vi "CenterBack.vi"(0 "Our Robot in":T3={"id"=0, "function"=enum."Attacker", "x"=0.0, "y"=0.0, "orientation"=0.0, "v_tangent"=0.0, "v_normal"=0.0, "v_ang"=0.0, "kick_x"=0.0, "kick_z"=0.0, "dribble"=FALSE, "Timestamp"=timestamp(0 s since 1904-01-01), "estimatives"={"est_v_tangent"=0.0, "est_v_normal"=0.0, "est_vx"=0.0, "est_vy"=0.0, "Pos Robot Est"=[]}, "dest_x_kick"=0.0, "dest_y_kick"=0.0, "Gap Coord"=[], "States"=enum."GoToTangent", "Path "=[], "Path  Smooth"=[], "Dest"=[]}, 1 "total":i32, 2 "Id duelist":u32, 3 "Stop?":bool, 4 "AI Parameters":T1={"GotoKick"={"Dist do cone a frente"=150.0, "attacker farback"=1500.0, "Perto"=300.0, "min dist to kick"=150.0, "kick eps"=0.05, "Time to transition"=0.0}, "Attacker"={"CC chute"=0.09, "CC passe"=0.045, "Kick Force"=100.0, "ball-robot Kick"=200.0, "ball-robot Pass"=0.3, "drible\nAttk"=FALSE}, "Defender"={"D max"=1700.0, "Vel p/ robô av"=1000.0, "Kick Force"=100.0, "D atk-def"=0.0, "D farback"=0.0, "drible\ndef"=FALSE, "drible\ngoalie"=FALSE}, "Timeout"={"Field/v in x"=6.0, "Dist Robots"=300, "Dist up in y"=300}, "Pose Striker"={"dist"=200.0, "Numeric"=-4.0, "dist 2"=200.0, "drible\nstriker"=FALSE}, "Dist Stop"=300.0, "D ball out"=200, "D central gap "=150.0, "T pass"=0.0, "Force ++"=0.0, "range kick"=0.0, "Chute alto"=TRUE, "Marcador novo"=TRUE, "drible"=FALSE, "D drible"=300.0} {"D drible" format="%#_13g"; "D central gap" format="%#_13g"; "Dist Stop" format="%#_13g"; "Pose Striker"."Numeric" format="%#_13g"; "Defender"."Kick Force" format="%#_13g"; "Defender"."Vel p/ robô av" format="%#_13g"; "Attacker"."ball-robot Kick" format="%#_13g"; "Attacker"."Kick Force" format="%#_13g"; "Attacker"."CC passe" format="%#_13g"; "Attacker"."CC chute" format="%#_13g"; "GotoKick"."kick eps" format="%#_13g"; "GotoKick"."min dist to kick" format="%#_13g"; "GotoKick"."Perto" format="%#_13g"; "GotoKick"."attacker farback" format="%#_13g"; "GotoKick"."Dist do cone a frente" format="%#_13g"}, 5 "balls":T8[](array[typedef]), 7 "Dribble":bool=TRUE, 9 "Field Size in":T9, 10 "Atacando contra?":bool=TRUE, 11 "Field defense":dbl[](array[numeric]), 12 "Defensores":u32[](array[numeric]), 14 "IA State Input 2":T2={"our_robots"=[], "enemy_robots"=[], "balls"=[], "geometry"={"line_width"=0, "field_length"=0, "field_width"=0, "boundary_width"=0, "referee_width"=0, "goal_width"=0, "goal_depth"=0, "goal_wall_width"=0, "center_circle_radius"=0, "defense_radius"=0, "defense_stretch"=0, "free_kick_from_defense_dist"=0, "penalty_spot_from_field_line_dist"=0, "penalty_line_from_spot_dist"=0}, "IA Judge"={"stage"="", "command"="", "our_goalie_id"=0.0, "enemy_goalie_id"=0.0, "command enum"=enum."Halt", "Time"=enum."Azul"}, "Received Timestamp"=timestamp(0 s since 1904-01-01), "Events"={"Touch"=FALSE, "Ball out"=FALSE, "id touch"=0.0, "Ball out of \nVision"=FALSE, "Ball inside \nGoalie area"=FALSE, "Robot not responding"=FALSE, "Robots responding status"=[1.0, 1.0, 1.0, 1.0, 1.0, 1.0], "Enemy Ball \nPossession"=FALSE, "Pass State"=FALSE, "id end of pass"=0.0, "Kick"=FALSE, "Id ini Possession"=0.0, "Ball Possesion"=FALSE, "Id Possesion"=0.0}}) -> (6 "Robot out":T3={"id"=0, "function"=enum."Attacker", "x"=0.0, "y"=0.0, "orientation"=0.0, "v_tangent"=0.0, "v_normal"=0.0, "v_ang"=0.0, "kick_x"=0.0, "kick_z"=0.0, "dribble"=FALSE, "Timestamp"=timestamp(0 s since 1904-01-01), "estimatives"={"est_v_tangent"=0.0, "est_v_normal"=0.0, "est_vx"=0.0, "est_vy"=0.0, "Pos Robot Est"=[]}, "dest_x_kick"=0.0, "dest_y_kick"=0.0, "Gap Coord"=[], "States"=enum."GoToTangent", "Path "=[], "Path  Smooth"=[], "Dest"=[]}, 8 "Pos Centers Back":dbl[][](array[numeric]), 13 "Zageuiro duelist?":bool=TRUE)   [LabVIEW 2017]
uses:
  Core/AI Robot.ctl
  Functions Enum.ctl
  AttackerStates.ctl
  Path Planning/RRT/PathDests.ctl
  Path Planning/RRT/PathDest.ctl
  Core/AI Ball.ctl
  Core/Field Size.ctl
  Core/AI Input.ctl
  Core/AI Judge.ctl
  Command Enum.ctl
  Util/Events/Events.ctl
  AI Parameters.ctl
  PersonalityEnum.ctl
  <vilib>/Analysis/_algsub.llb/Real Vector Norm.vi
  <vilib>/Analysis/NI_AALPro.lvlib
panel:
  in  "element":dbl=-2000.0 format="%#_13g"
  in  "dist to defender\nattacker evasion":dbl=200.0
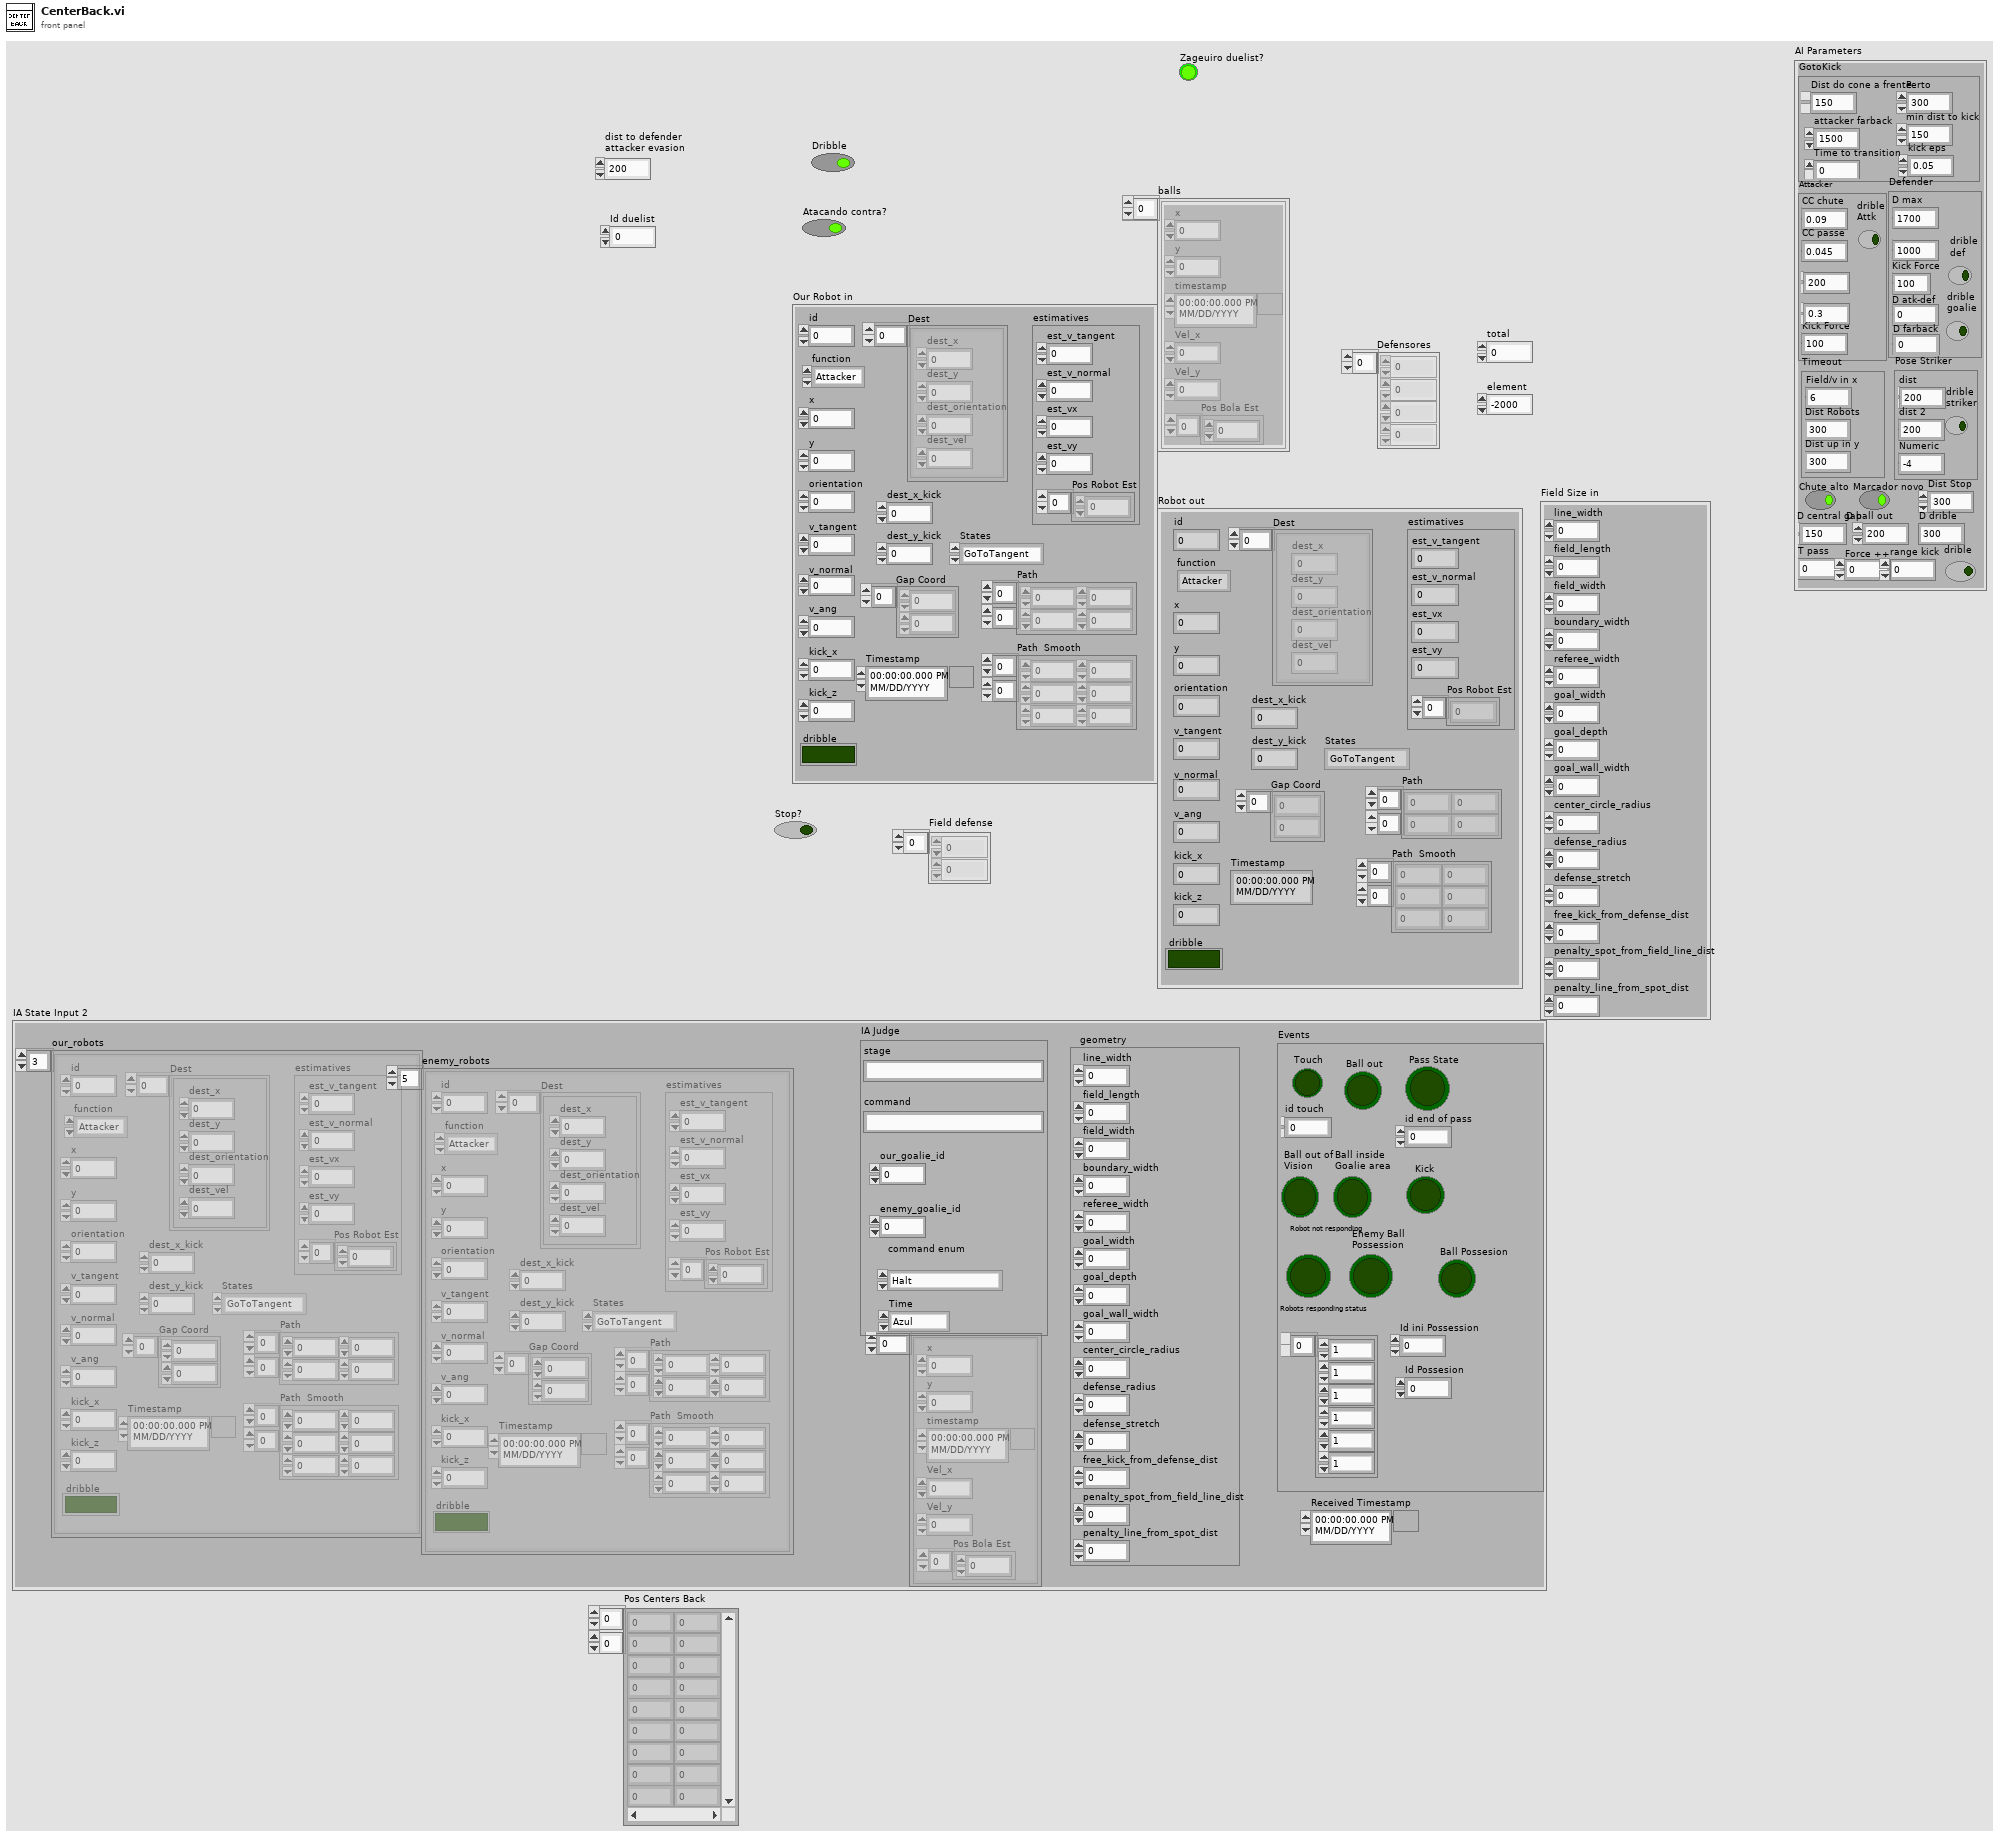
[diagram p1: front panel]
types:
  T1 = typedef "AI Parameters.ctl" = cluster{"GotoKick":cluster{"Dist do cone a frente":dbl, "attacker farback":dbl, "Perto":dbl, "min dist to kick":dbl, "kick eps":dbl, "Time to transition":dbl}, "Attacker":cluster{"CC chute":dbl, "CC passe":dbl, "Kick Force":dbl, "ball-robot Kick":dbl, "ball-robot Pass":dbl, "drible\nAttk":bool}, "Defender":cluster{"D max":dbl, "Vel p/ robô av":dbl, "Kick Force":dbl, "D atk-def":dbl, "D farback":dbl, "drible\ndef":bool, "drible\ngoalie":bool}, "Timeout":cluster{"Field/v in x":dbl, "Dist Robots":u32, "Dist up in y":u32}, "Pose Striker":cluster{"dist":dbl, "Numeric":dbl, "dist 2":dbl, "drible\nstriker":bool}, "Dist Stop":dbl, "D ball out":i32, "D central gap ":dbl, "T pass":dbl, "Force ++":dbl, "range kick":dbl, "Chute alto":bool, "Marcador novo":bool, "drible":bool, "D drible":dbl}
  T2 = typedef "AI Input.ctl" = cluster{"our_robots":T3[], "enemy_robots":T3[], "balls":T8[], "geometry":T9, "IA Judge":T10, "Received Timestamp":timestamp, "Events":T12}
  T3 = typedef "AI Robot.ctl" = cluster{"id":u32, "function":T4, "x":dbl, "y":dbl, "orientation":dbl, "v_tangent":dbl, "v_normal":dbl, "v_ang":dbl, "kick_x":dbl, "kick_z":dbl, "dribble":bool, "Timestamp":timestamp, "estimatives":cluster{"est_v_tangent":dbl, "est_v_normal":dbl, "est_vx":dbl, "est_vy":dbl, "Pos Robot Est":dbl[]}, "dest_x_kick":dbl, "dest_y_kick":dbl, "Gap Coord":dbl[], "States":T5, "Path ":dbl[][], "Path  Smooth":dbl[][], "Dest":T6}
  T4 = typedef "Functions Enum.ctl" = enum16{"Attacker", "Goalie", "Defender", "Striker", "Goto 0", "Dummy", "Kicker", "ZigZag"}
  T5 = typedef "AttackerStates.ctl" = enum16{"Pass", "GoToTangent", "BallGetting", "GoToKick", ""}
  T6 = typedef "PathDests.ctl" = T7[]
  T7 = typedef "PathDest.ctl" = cluster{"dest_x":dbl, "dest_y":dbl, "dest_orientation":dbl, "dest_vel":dbl}
  T8 = typedef "AI Ball.ctl" = cluster{"x":dbl, "y":dbl, "timestamp":timestamp, "Vel_x":dbl, "Vel_y":dbl, "Pos Bola Est":dbl[]}
  T9 = typedef "Field Size.ctl" = cluster{"line_width":u32, "field_length":u32, "field_width":u32, "boundary_width":u32, "referee_width":u32, "goal_width":u32, "goal_depth":u32, "goal_wall_width":u32, "center_circle_radius":u32, "defense_radius":u32, "defense_stretch":u32, "free_kick_from_defense_dist":u32, "penalty_spot_from_field_line_dist":u32, "penalty_line_from_spot_dist":u32}
  T10 = typedef "AI Judge.ctl" = cluster{"stage":string, "command":string, "our_goalie_id":dbl, "enemy_goalie_id":dbl, "command enum":T11, "Time":enum16{"Azul", "Amarelo"}}
  T11 = typedef "Command Enum.ctl" = enum16{"Halt", "Stop", "Force Start", "PKA Normal Start", "Prepare Kickoff Ally", "PKE Normal Start", "Prepare Kickoff Enemy", "Prepare Penalty Ally", "PPA Normal Start", "Prepare Penalty Enemy", "PPE Normal Start", "Direct Free Enemy", "Direct Free Ally", "Indirect Free Enemy", "Indirect Free Ally", "Timeout Enemy", "Timeout Ally", "Goal Enemy", "Goal Ally", "Ball Placement Enemy", "Ball Placement Ally", "Normal Half Time", "Extra Time Break", "Extra Half Time", "None", "Post Game"}
  T12 = typedef "Events.ctl" = cluster{"Touch":bool, "Ball out":bool, "id touch":dbl, "Ball out of \nVision":bool, "Ball inside \nGoalie area":bool, "Robot not responding":bool, "Robots responding status":dbl[], "Enemy Ball \nPossession":bool, "Pass State":bool, "id end of pass":dbl, "Kick":bool, "Id ini Possession":dbl, "Ball Possesion":bool, "Id Possesion":dbl}
  T13 = cluster{"D max":dbl, "Vel p/ robô av":dbl, "Kick Force":dbl, "D atk-def":dbl, "D farback":dbl, "drible\ndef":bool, "drible\ngoalie":bool}
  T14 = typedef "PersonalityEnum.ctl" = enum16{"Attacker", "Striker", "Defender", "Goalie"}
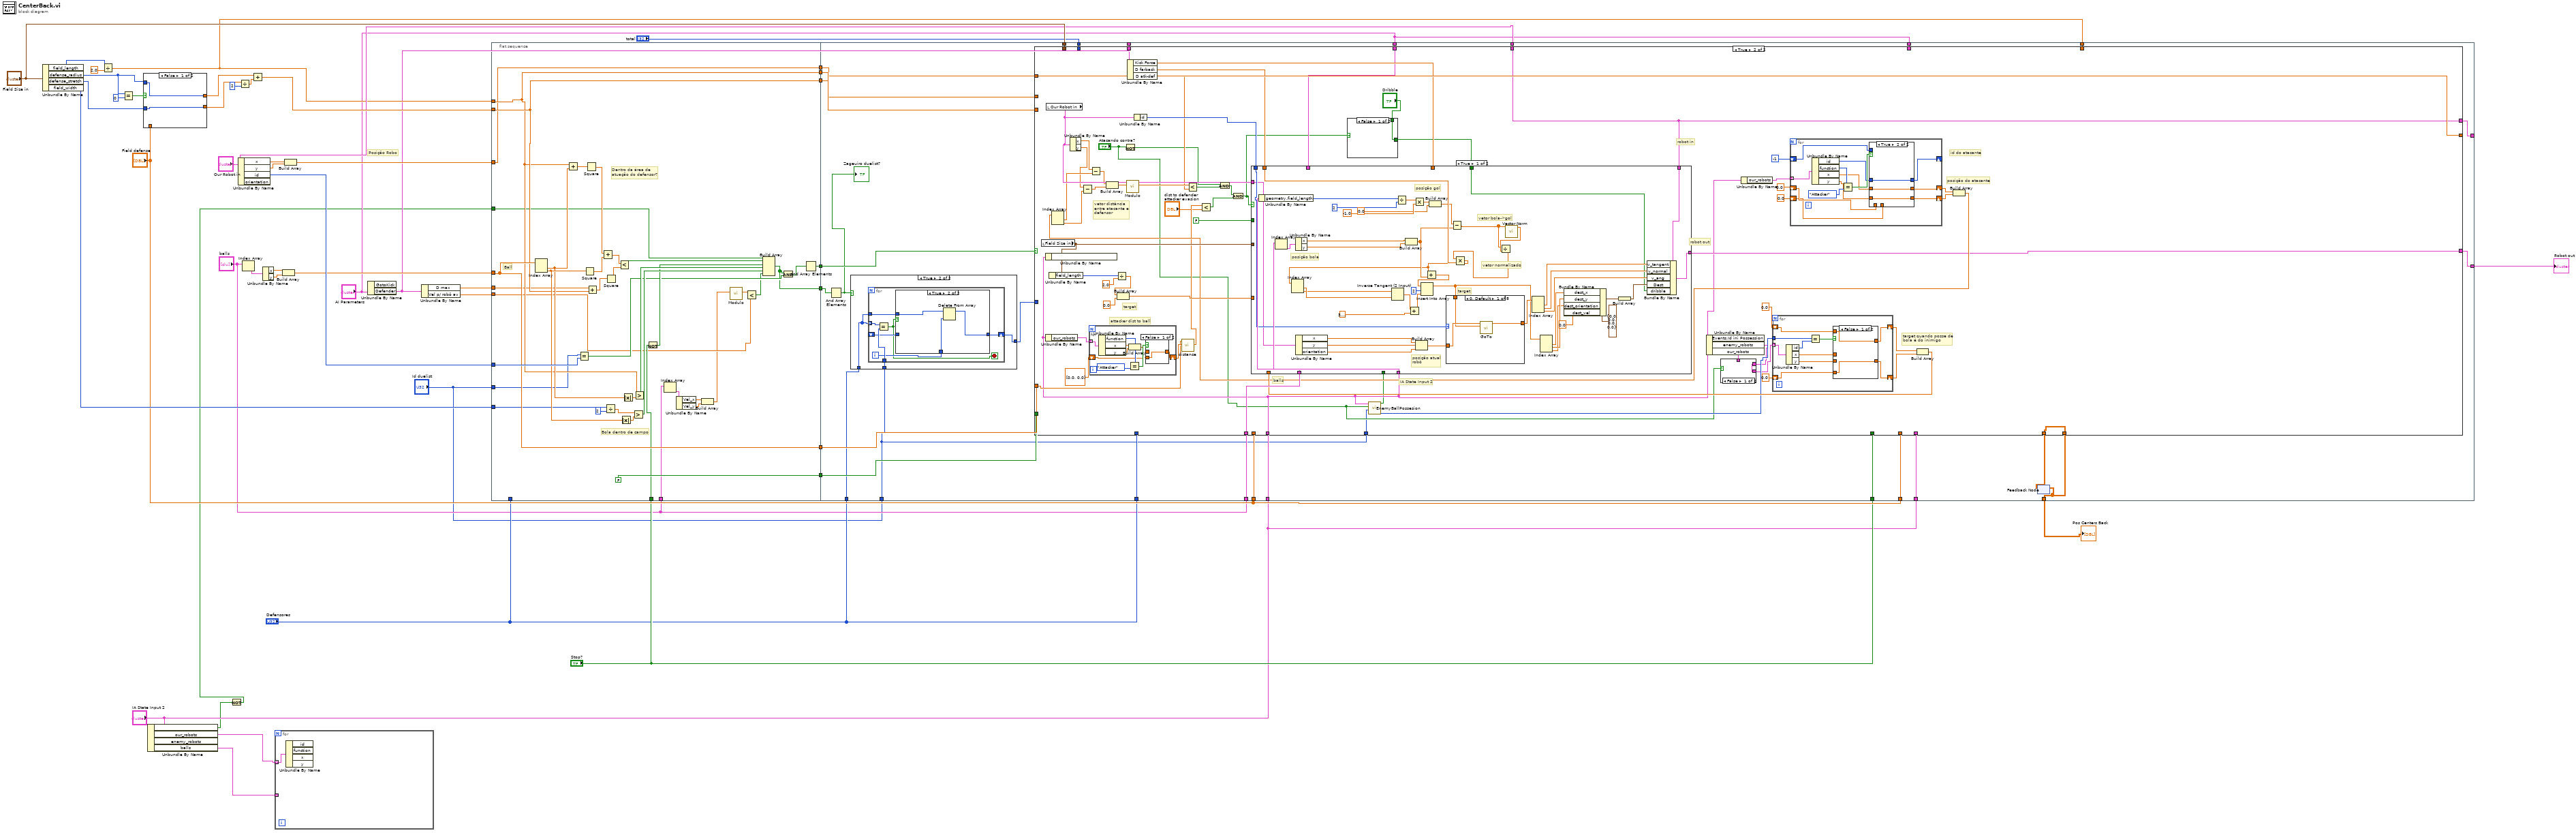
[diagram p0: block diagram]
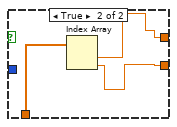
[diagram p2: hidden frame]
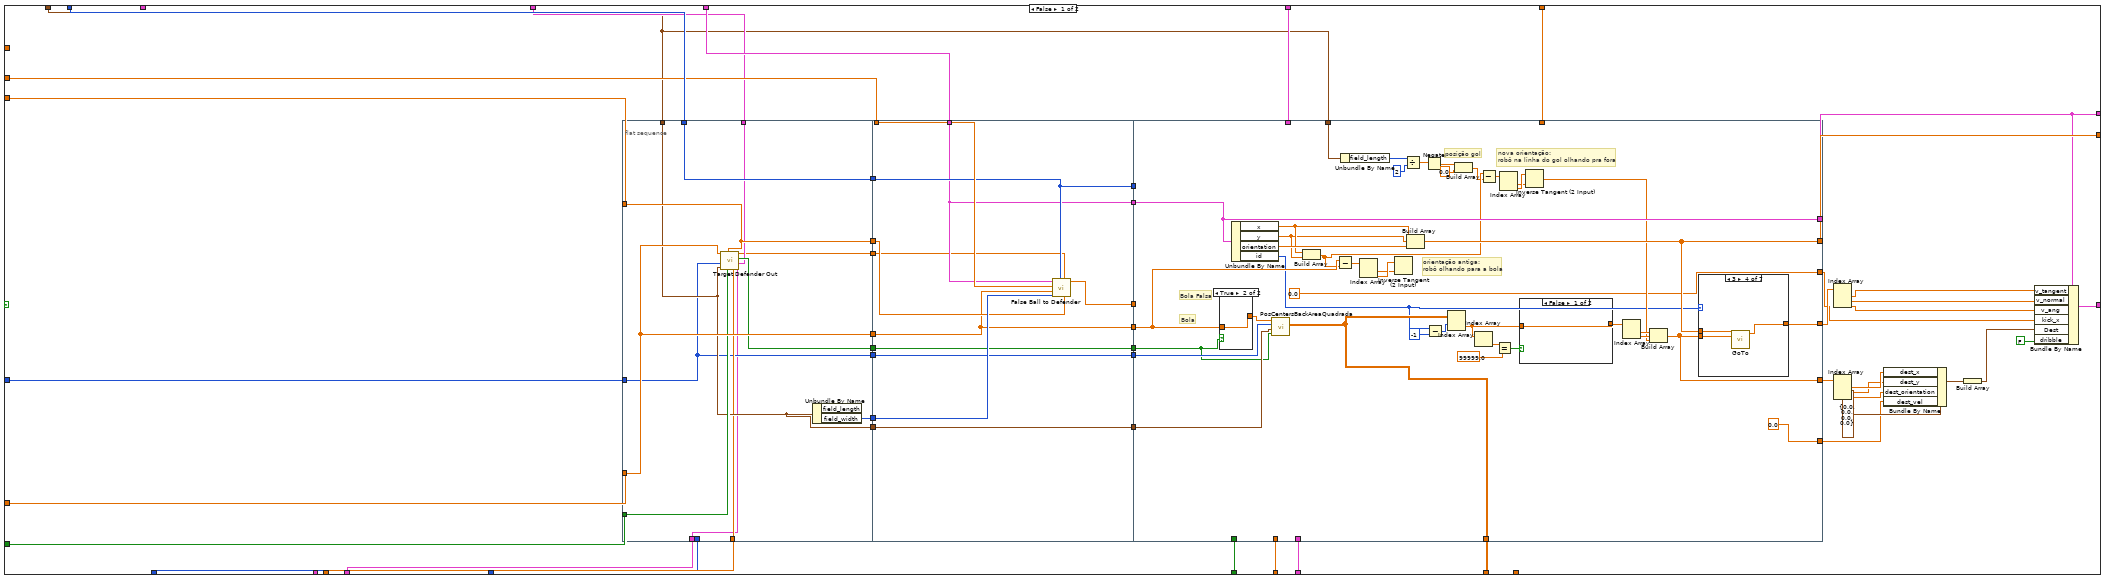
[diagram p5: hidden frame]
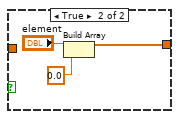
[diagram p6: hidden frame]
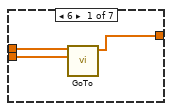
[diagram p7: hidden frame]
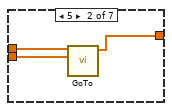
[diagram p8: hidden frame]
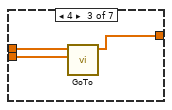
[diagram p9: hidden frame]
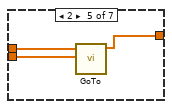
[diagram p10: hidden frame]
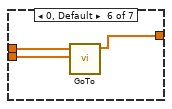
[diagram p11: hidden frame]
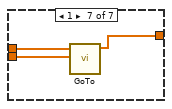
[diagram p12: hidden frame]
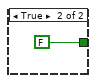
[diagram p14: hidden frame]
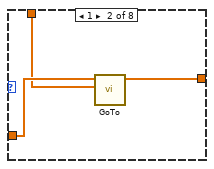
[diagram p17: hidden frame]
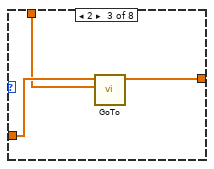
[diagram p18: hidden frame]
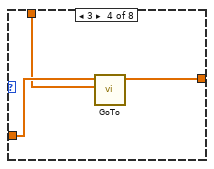
[diagram p19: hidden frame]
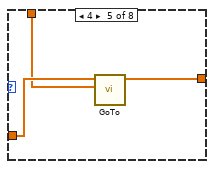
[diagram p20: hidden frame]
diagram:
  # "Posição Robo"
  n1 = Unbundle By Name("Field Size in") -> ("field_length"=w42:u32, "defense_radius"=w26:u32, "defense_stretch"=w25:u32, "field_width"=w39:u32)
  n2 = Divide(x=w42, y=2.0) -> (x/y=w17:dbl)
  n3 = Equal?(x=w26, y=u32 0) -> (x = y?=w24:bool)
  n4 = case shown="False" w24 {
    tunnel: [w49 w51] -> w23
    tunnel: w26 -> [w49 _]
    tunnel: w25 -> [w48 _]
    tunnel: [w48 w50] -> w22
    tunnel: "Field defense" -> [_ w52]
    frame False {
    }
    frame True {
      n5 = Index Array(array=w52) -> (element #1=w51:dbl, element #2=w50:dbl)  [unwired: 2 in]
    }
  }
  n6 = Unbundle By Name("IA State Input 2") -> ("Events.Ball inside \nGoalie area"=w2:bool, "our_robots"=w7:T3[], "balls"=w6:T8[])  [unwired: 1 out]
  n7 = Not(x=w2) -> (.not. x?=w1:bool)
  n8 = Unbundle By Name("Our Robot in") -> ("x"=w36:dbl, "y"=w35:dbl, "id"=w40:u32)  [unwired: 1 out]
  n9 = Divide(x=w22, y=u32 2) -> (x/y=w46:dbl)
  n10 = Index Array(array="balls") -> (element=w47:T8)  [unwired: 1 in]
  n11 = Add(x=w23, y=w46) -> (x+y=w41:dbl)
  n12 = Unbundle By Name(w47) -> ("x"=w44:dbl, "y"=w9:dbl)
  n13 = for {
    tunnel: w7 -> [w53] mode=indexing
    tunnel: w6 -> [_] mode=indexing
    n14 = Unbundle By Name(w53) -> ()  [unwired: 4 out]
  }
  n15 = Build Array(w44, w9) -> (w18:dbl[])
  n16 = Build Array(w36, w35) -> (w19:dbl[])
  n17 = Unbundle By Name("AI Parameters") -> ("Defender"=w11:T13)  [unwired: 1 out]
  n18 = Unbundle By Name(w11) -> ("D max"=w13:dbl, "Vel p/ robô av"=w12:dbl)
  n19 = flat-sequence {
    tunnel: w41 -> [w72]
    tunnel: w17 -> [w71]
    tunnel: w18 -> [w87]
    tunnel: w19 -> [w70]
    tunnel: [w87] -> w34
    tunnel: [w92] -> w33
    tunnel: w40 -> [w91]
    tunnel: w39 -> [w78]
    tunnel: [FALSE ("Target Fora")] -> w32
    tunnel: [w71] -> w31
    tunnel: [w72] -> w30
    tunnel: [w70] -> w29
    tunnel: "Defensores" -> [_]
    tunnel: "Stop?" -> [w69]
    tunnel: [w65] -> w15
    tunnel: "balls" -> [w64]
    tunnel: w13 -> [w61]
    tunnel: w12 -> [w60]
    tunnel: "Id duelist" -> [w55]
    tunnel: w1 -> [w54]
    tunnel: "total" -> [w121]
    tunnel: [w120] -> w5
    tunnel: w34 -> [w119]
    tunnel: w33 -> [w118]
    tunnel: w32 -> [w117]
    tunnel: w31 -> [w115]
    tunnel: "Field Size in" -> [w116]
    tunnel: "Our Robot in" -> [w114]
    tunnel: w30 -> [w113]
    tunnel: [w112] -> _
    tunnel: w29 -> [w111]
    tunnel: "Field defense" -> [w110]
    tunnel: "Field defense" -> [w109]
    tunnel: "Defensores" -> [w108]
    tunnel: "IA State Input 2" -> [w107]
    tunnel: "balls" -> [w106]
    tunnel: "Stop?" -> [w105]
    tunnel: w17 -> [w104]
    tunnel: "Defensores" -> [w103]
    tunnel: w15 -> [w102]
    tunnel: w11 -> [w100]
    tunnel: "AI Parameters" -> [w99]
    tunnel: "AI Parameters" -> [w98]
    tunnel: "IA State Input 2" -> [w97]
    tunnel: [w94] -> w4
    tunnel: "Id duelist" -> [w93]
    frame #0 {
      # "Bola dentro de campo"
      # "Dentro da área de \natuação do defensor?"
      # "Ball"
      n20 = Index Array(array=w87) -> (element #1=w75:dbl, element #2=w79:dbl)  [unwired: 2 in]
      n21 = Add(x=w71, y=w75) -> (x+y=w88:dbl)
      n22 = Equal?(x=w55, y=w91) -> (x = y?=w67:bool)
      n23 = Square(x=w79) -> (x^2=w90:dbl)
      n24 = Square(x=w88) -> (x^2=w89:dbl)
      n25 = Add(x=w61, y=w72) -> (x+y=w74:dbl)
      n26 = Add(x=w89, y=w90) -> (x+y=w84:dbl)
      n27 = Divide(x=w78, y=u32 2) -> (x/y=w81:dbl)
      n28 = Square(x=w74) -> (x^2=w86:dbl)
      n29 = Less?(x=w84, y=w86) -> (x < y?=w85:bool)
      n30 = Absolute Value(x=w79) -> (abs(x)=w80:dbl)
      n31 = Absolute Value(x=w75) -> (abs(x)=w83:dbl)
      n32 = Greater?(x=w81, y=w80) -> (0:w76:bool)
      n33 = Greater?(x=w71, y=w83) -> (0:w82:bool)
      n34 = Not(x=w69) -> (.not. x?=w68:bool)
      n35 = Index Array(array=w64) -> (element=w59:T8)  [unwired: 1 in]
      n36 = Unbundle By Name(w59) -> ("Vel_x"=w58:dbl, "Vel_y"=w57:dbl)
      n37 = Build Array(w58, w57) -> (w56:dbl[])
      n38 = call "Modulo.vi"("2D vector"=w56) -> ("Modulo"=w62:dbl)  [unwired: 10 in]
      n39 = Less?(x=w62, y=w60) -> (x < y?=w63:bool)
      n40 = Build Array(w54, w85, w68, w82, w76, w63) -> (w65:bool[])
      n41 = And(x=w65, y=w67) -> (x .and. y?=w66:bool[])
      n42 = And Array Elements(Boolean array=w66) -> (logical AND=w92:bool)
    }
    frame #1 {
      n43 = And Array Elements(Boolean array=w102) -> (logical AND=w96:bool)
      "Zageuiro duelist?" <- w96
      n44 = case shown="True" w96 {
        tunnel: w103 -> [w122 w124]
        tunnel: [w122 w123] -> w101
        tunnel: w93 -> [_ w125]
        frame False {
        }
        frame True {
          n45 = for {
            tunnel: w124 -> [w132] mode=indexing
            tunnel: w125 -> [w131]
            tunnel: w124 -> [w130]
            shift-right: [w128] -> w123
            shift-left: _ -> [w127]
            i -> [w129]
            stop <- w126 stop-if-true
            n46 = Equal?(x=w132, y=w131) -> (x = y?=w126:bool)
            n47 = case shown="True" w126 {
              tunnel: w130 -> [_ w136]
              tunnel: w129 -> [_ w135]
              tunnel: [w133 w134] -> w128
              tunnel: w127 -> [w133 _]
              frame False {
              }
              frame True {
                n48 = Delete From Array(array=w136, index=w135) -> (array with subset deleted=w134:u32[])  [unwired: 1 in, 1 out]
              }
            }
          }
        }
      }
      n49 = feedback #1() -> (w94:dbl[][])  [unwired: 1 in]
      n50 = case shown="True" w118 {
        tunnel: w121 -> [w185 _]
        tunnel: [w181 w301] -> w120
        tunnel: w119 -> [w180 w294]
        tunnel: w117 -> [w178 _]
        tunnel: w115 -> [w177 _]
        tunnel: w116 -> [w147 _]
        tunnel: w114 -> [w176 w302]
        tunnel: w113 -> [w175 _]
        tunnel: [w161 w336] -> _
        tunnel: [w160 w302] -> w112
        tunnel: w111 -> [_ w336]
        tunnel: w110 -> [w159 _]
        tunnel: w109 -> [w158 _]
        tunnel: w108 -> [w157 _]
        tunnel: w107 -> [w150 w288]
        tunnel: w106 -> [_ w335]
        tunnel: w105 -> [w156 _]
        tunnel: w104 -> [w155 _]
        tunnel: w101 -> [w153 _]
        tunnel: w100 -> [_ w321]
        tunnel: w99 -> [w149 w319]
        tunnel: w98 -> [w152 _]
        tunnel: w97 -> [w151 _]
        tunnel: [w140 w289] -> w95
        tunnel: w94 -> [_ w289]
        tunnel: w93 -> [_ w280]
        frame False {
          n51 = flat-sequence {
            tunnel: w185 -> [w197]
            tunnel: [w198] -> w186
            tunnel: w180 -> [w196]
            tunnel: [w197] -> w179
            tunnel: w178 -> [w194]
            tunnel: w177 -> [w195]
            tunnel: w147 -> [w192]
            tunnel: [w196] -> w174
            tunnel: [w195] -> w173
            tunnel: [w193] -> w169
            tunnel: [w190] -> w166
            tunnel: [w192] -> w164
            tunnel: w158 -> [w191]
            tunnel: w157 -> [_]
            tunnel: w153 -> [w190]
            tunnel: w150 -> [w189]
            tunnel: w149 -> [w188]
            tunnel: [w187] -> w148
            tunnel: w186 -> [w209]
            tunnel: w179 -> [w204]
            tunnel: w176 -> [w201]
            tunnel: w175 -> [w208]
            tunnel: w174 -> [w206]
            tunnel: w173 -> [w207]
            tunnel: [w199] -> w172
            tunnel: [w206] -> w171
            tunnel: [w205] -> w170
            tunnel: w169 -> [w205]
            tunnel: [w204] -> w168
            tunnel: [w203] -> w167
            tunnel: w166 -> [w203]
            tunnel: [w202] -> w165
            tunnel: w164 -> [w202]
            tunnel: [w201] -> w163
            tunnel: w148 -> [w200]
            tunnel: [w243] -> w162
            tunnel: [w242] -> w160
            tunnel: w172 -> [_]
            tunnel: w171 -> [w238]
            tunnel: w170 -> [w210]
            tunnel: w168 -> [_]
            tunnel: w167 -> [w216]
            tunnel: w165 -> [w217]
            tunnel: w163 -> [w242]
            tunnel: [w239] -> w161
            tunnel: w159 -> [_]
            tunnel: w156 -> [_]
            tunnel: w155 -> [_]
            tunnel: [w232] -> w154
            tunnel: w152 -> [_]
            tunnel: w151 -> [_]
            tunnel: w147 -> [w231]
            tunnel: [w214] -> w140
            tunnel: [0.0 ("dest_vel")] -> w139
            tunnel: [0.0 ("kick_x")] -> w138
            frame #0 {
              n52 = call "Target Defender Out.vi"("IA State Input"=w189, "AI Parameters"=w188, "Field defense"=w191, "Target Fora in"=w194, "Campo/2"=w195, "Field Size in"=w192, "Defensores"=w190, "Ball"=w196) -> ("Target Fora out"=w193:bool, "Central Position"=w187:dbl[])  [unwired: 2 in]
              n53 = Unbundle By Name(w192) -> ("field_width"=w198:u32)  [unwired: 1 out]
            }
            frame #1 {
              n54 = call "False Ball to Defender.vi"("Campo/2"=w207, "Central Position"=w200, "field_width"=w209, "total"=w204, "Bola"=w206, "raio da área \ndo goleiro"=w208, "Our Robot in"=w201) -> ("Bola Falsa"=w199:dbl[])  [unwired: 4 in]
            }
            frame #2 {
              # "nova orientação:\nrobô na linha do gol olhando pra fora"
              # "orientação antiga:\nrobô olhando para a bola"
              # "posição gol"
              # "Bola"
              # "Bola Falsa"
              n55 = case shown="True" w210 {
                tunnel: [w275 w276] -> w215
                tunnel: w238 -> [w275 w276]
                frame False {
                }
                frame True {
                }
              }
              n56 = Unbundle By Name(w242) -> ("x"=w248:dbl, "y"=w247:dbl, "orientation"=w249:dbl, "id"=w213:u32)
              n57 = call "PosCentersBackAreaQuadrada.vi"("Robô fora?"=w210, "geometry"=w217, "Defensores"=w216, "Pos Bola"=w215) -> ("Pos Centers Back"=w214:dbl[][])  [unwired: 6 in, 1 out]
              n58 = Build Array(w248, w247) -> (w225:dbl[])
              n59 = Subtract(x=w238, y=w225) -> (x-y=w246:dbl[])
              n60 = Unbundle By Name(w231) -> ("field_length"=w230:u32)
              n61 = Index Array(array=w246) -> (element #1=w244:dbl, element #2=w245:dbl)  [unwired: 2 in]
              n62 = Inverse Tangent (2 Input)(1:w244, 2:w245) -> ()  [unwired: 1 out]
              n63 = Divide(x=w230, y=u32 2) -> (x/y=w228:dbl)
              n64 = Build Array(w248, w247, w249) -> (w239:dbl[])
              n65 = Negate(x=w228) -> (-x=w227:dbl)
              n66 = Subtract(x=w213, y=-1) -> (x-y=w211:u32)
              n67 = Index Array(array=w214, index (row)=w211) -> (element=w236:dbl[])  [unwired: 1 in]
              n68 = Build Array(w227, 0.0 ("element")) -> (w224:dbl[])
              n69 = Index Array(array=w236) -> (element=w235:dbl)  [unwired: 1 in]
              n70 = Subtract(x=w225, y=w224) -> (x-y=w223:dbl[])
              n71 = Equal?(x=w235, y=99999.0) -> (x = y?=w234:bool)
              n72 = Index Array(array=w223) -> (element #1=w221:dbl, element #2=w222:dbl)  [unwired: 2 in]
              n73 = case shown="False" w234 {
                tunnel: [w250 w252] -> w237
                tunnel: w236 -> [w250 _]
                frame False {
                }
                frame True {
                  n74 = Build Array("element", 0.0 ("element")) -> (w252:dbl[])
                }
              }
              n75 = Inverse Tangent (2 Input)(1:w221, 2:w222) -> (0:w220:dbl)
              n76 = Index Array(array=w237) -> (element #1=w241:dbl, element #2=w240:dbl)  [unwired: 2 in]
              n77 = Build Array(w241, w240, w220) -> (w232:dbl[])
              n78 = case shown="3" w213 {
                tunnel: [w254 w257 w260 w263 w266 w269 w272] -> w243
                tunnel: w232 -> [w255 w259 w261 w264 w267 w270 w273]
                tunnel: w239 -> [w256 w258 w262 w265 w268 w271 w274]
                frame 6 {
                  n79 = call "GoTo.vi"("Target"=w255, "Position"=w256) -> ("Output\nVelocity"=w254:dbl[])  [unwired: 8 in, 1 out]
                }
                frame 5 {
                  n80 = call "GoTo.vi"("Target"=w259, "Position"=w258) -> ("Output\nVelocity"=w257:dbl[])  [unwired: 8 in, 1 out]
                }
                frame 4 {
                  n81 = call "GoTo.vi"("Target"=w261, "Position"=w262) -> ("Output\nVelocity"=w260:dbl[])  [unwired: 8 in, 1 out]
                }
                frame 3 {
                  n82 = call "GoTo.vi"("Target"=w264, "Position"=w265) -> ("Output\nVelocity"=w263:dbl[])  [unwired: 8 in, 1 out]
                }
                frame 2 {
                  n83 = call "GoTo.vi"("Target"=w267, "Position"=w268) -> ("Output\nVelocity"=w266:dbl[])  [unwired: 8 in, 1 out]
                }
                frame 0, Default {
                  n84 = call "GoTo.vi"("Target"=w270, "Position"=w271) -> ("Output\nVelocity"=w269:dbl[])  [unwired: 8 in, 1 out]
                }
                frame 1 {
                  n85 = call "GoTo.vi"("Target"=w273, "Position"=w274) -> ("Output\nVelocity"=w272:dbl[])  [unwired: 8 in, 1 out]
                }
              }
            }
          }
          n86 = Index Array(array=w162) -> (element #1=w184:dbl, element #2=w183:dbl, element #3=w182:dbl)  [unwired: 3 in]
          n87 = Index Array(array=w154) -> (element #1=w143:dbl, element #2=w142:dbl, element #3=w141:dbl)  [unwired: 3 in]
          n88 = Bundle By Name(cluster=T7 {"dest_x"=0.0, "dest_y"=0.0, "dest_orientation"=0.0, "dest_vel"=0.0} ("Dest"), "dest_x"=w143, "dest_y"=w142, "dest_orientation"=w141, "dest_vel"=w139) -> (w145:T7)
          n89 = Build Array(w145) -> (w144:T7[])
          n90 = Bundle By Name(cluster=w160, "v_tangent"=w184, "v_normal"=w183, "v_ang"=w182, "kick_x"=w138, "Dest"=w144, "dribble"=FALSE) -> (w181:T3)
        }
        frame True {
          # "attacker dist to ball"
          # "robot in"
          # "vetor distância\nentre atacante e \ndefensor"
          # "posição do atacante"
          # "id do atacante"
          # "target quando posse de\nbola é do inimigo"
          # "target"
          # "balls"
          # "IA State Input 2"
          # "robot out"
          n91 = local read "Field Size in"() -> (w331:T9)
          n92 = Unbundle By Name(w288) -> ()  [unwired: 1 out]
          n93 = Unbundle By Name(w288) -> ("our_robots"=w297:T3[])
          n94 = local read "Our Robot in"() -> (w312:T3)
          n95 = Unbundle By Name(w331) -> ("field_length"=w330:u32)
          n96 = Unbundle By Name(w312) -> ("x"=w310:dbl, "y"=w308:dbl)
          n97 = for {
            tunnel: w297 -> [w349] mode=indexing
            shift-right: [w343] -> w295
            shift-left: dbl[] [0.0, 0.0] -> [w342]
            n98 = Unbundle By Name(w349) -> ("function"=w348:T4, "x"=w341:dbl, "y"=w345:dbl)
            n99 = Build Array(w341, w345) -> (w344:dbl[])
            n100 = Equal?(x=w348, y=Functions_Enum."Attacker") -> (x = y?=w346:bool)
            n101 = case shown="False" w346 {
              tunnel: w344 -> [_ w351]
              tunnel: [w350 w351] -> w343
              tunnel: w342 -> [w350 _]
              frame False {
              }
              frame True {
              }
            }
          }
          n102 = Divide(x=w330, y=2.0) -> (x/y=w328:dbl)
          n103 = Build Array(w328, 0.0) -> (w333:dbl[])
          n104 = Not(x="Atacando contra?") -> (.not. x?=w285:bool)
          n105 = Unbundle By Name(w321) -> ("Kick Force"=w320:dbl, "D farback"=w299:dbl, "D atk-def"=w300:dbl)
          n106 = Unbundle By Name(w312) -> ("id"=w334:u32)
          n107 = call "distance.vi"("target pos"=w295, "obj pos"=w294) -> ("sqrt(x)"=w293:dbl)  [unwired: 9 in]
          n108 = Less?(x=w293, y="dist to defender\nattacker evasion") -> (x < y?=w291:bool)
          n109 = call "EnemyBallPossesion.vi"("Id Duelist"=w280, "Atacando contra?"="Atacando contra?", "IA State Input"=w288) -> ("Id Enemy Ball Possesion"=w287:u32, "Enemy Ball Possesion?"=w286:bool)  [unwired: 7 in]
          n110 = Unbundle By Name(w288) -> ("enemy_robots"=w281:T3[], "our_robots"=w282:T3[])  [unwired: 1 out]
          n111 = case shown="False" "Atacando contra?" {
            tunnel: [w339 w340] -> w283
            tunnel: w282 -> [_ w340]
            tunnel: w281 -> [w339 _]
            frame False {
            }
            frame True {
            }
          }
          n112 = Unbundle By Name(w288) -> ("our_robots"=w318:T3[])
          n113 = for {
            tunnel: w283 -> [w576] mode=indexing
            tunnel: w287 -> [w574]
            shift-right: [w570] -> w326
            shift-left: 0.0 ("x") -> [w568]
            shift-right: [w569] -> w325
            shift-left: 0.0 ("y") -> [w567]
            n114 = Unbundle By Name(w576) -> ("id"=w575:u32, "x"=w572:dbl, "y"=w571:dbl)
            n115 = Equal?(x=w574, y=w575) -> (x = y?=w573:bool)
            n116 = case shown="False" w573 {
              tunnel: w572 -> [_ w580]
              tunnel: w571 -> [_ w579]
              tunnel: [w578 w580] -> w570
              tunnel: [w577 w579] -> w569
              tunnel: w568 -> [w578 _]
              tunnel: w567 -> [w577 _]
              frame False {
              }
              frame True {
              }
            }
          }
          n117 = for {
            tunnel: w318 -> [w560] mode=indexing
            shift-right: [w553] -> _
            shift-left: -1 -> [w552]
            shift-right: [w551] -> w314
            shift-left: 0.0 ("y") -> [w549]
            shift-right: [w550] -> w313
            shift-left: 0.0 ("y") -> [w548]
            n118 = Unbundle By Name(w560) -> ("id"=w556:u32, "function"=w559:T4, "x"=w555:dbl, "y"=w554:dbl)
            n119 = Equal?(x=w559, y=Functions_Enum."Attacker" ("x")) -> (x = y?=w557:bool)
            n120 = case shown="True" w557 {
              tunnel: w556 -> [_ w564]
              tunnel: w555 -> [_ w566]
              tunnel: w554 -> [_ w565]
              tunnel: [w562 w566] -> w551
              tunnel: [w561 w565] -> w550
              tunnel: [w563 w564] -> w553
              tunnel: w552 -> [w563 _]
              tunnel: w549 -> [w562 _]
              tunnel: w548 -> [w561 _]
              frame False {
              }
              frame True {
              }
            }
          }
          n121 = Build Array(w326, w325) -> (w322:dbl[])
          n122 = Build Array(w314, w313) -> (w311:dbl[])
          n123 = Index Array(array=w311) -> (element #1=w309:dbl, element #2=w307:dbl)  [unwired: 2 in]
          n124 = Subtract(x=w308, y=w307) -> (x-y=w305:dbl)
          n125 = Subtract(x=w310, y=w309) -> (x-y=w306:dbl)
          n126 = Build Array(w306, w305) -> (w304:dbl[])
          n127 = call "Modulo.vi"("2D vector"=w304) -> ("Modulo"=w303:dbl)  [unwired: 10 in]
          n128 = Less?(x=w303, y=w300) -> (x < y?=w298:bool)
          n129 = And(x=w285, y=w298) -> (x .and. y?=w290:bool)
          n130 = And(x=w290, y=w291) -> (x .and. y?=w279:bool)
          n131 = case shown="False" w279 {
            tunnel: [w337 FALSE] -> w278
            tunnel: "Dribble" -> [w337 _]
            frame False {
            }
            frame True {
            }
          }
          n132 = case shown="True" w279 {
            tunnel: w335 -> [w391 w435]
            tunnel: w334 -> [w386 w434]
            tunnel: w333 -> [_ w426]
            tunnel: w331 -> [_ w433]
            tunnel: FALSE -> [_ w432]
            tunnel: w322 -> [_ w427]
            tunnel: w320 -> [_ w431]
            tunnel: w319 -> [_ w430]
            tunnel: w288 -> [w392 w423]
            tunnel: w312 -> [w385 w429]
            tunnel: w302 -> [w372 _]
            tunnel: [w371 w428] -> w301
            tunnel: w299 -> [w369 _]
            tunnel: w278 -> [w352 w424]
            tunnel: w286 -> [_ w422]
            frame True {
              # "target"
              # "posição atual\nrobô"
              # "vetor normalizado"
              # "vetor bola->gol"
              # "posição bola"
              # "posição gol"
              n133 = Unbundle By Name(w392) -> ("geometry.field_length"=w393:u32)
              n134 = Index Array(array=w391) -> (element=w397:T8)  [unwired: 1 in]
              n135 = Unbundle By Name(w397) -> ("x"=w366:dbl, "y"=w365:dbl)
              n136 = Unbundle By Name(w385) -> ("x"=w384:dbl, "y"=w383:dbl, "orientation"=w382:dbl)
              n137 = Divide(x=w393, y=u32 2) -> (x/y=w395:dbl)
              n138 = Build Array(w366, w365) -> (w362:dbl[])
              n139 = Multiply(x=w395, y=-1.0) -> (x*y=w368:dbl)
              n140 = Build Array(w384, w383, w382) -> (w381:dbl[])
              n141 = Build Array(w368, 0.0 ("element")) -> (w364:dbl[])
              n142 = Subtract(x=w364, y=w362) -> (x-y=w363:dbl[])
              n143 = call-poly <vilib>:"Vector Norm.vi"("Input Vector"=w363) -> ("norm"=w390:dbl)  [unwired: 9 in, 1 out]
              n144 = Divide(x=w363, y=w390) -> (x/y=w370:dbl[])
              n145 = Multiply(x=w370, y=w369) -> (x*y=w360:dbl[])
              n146 = Index Array(array=w360) -> (element #1=w389:dbl, element #2=w388:dbl)  [unwired: 2 in]
              n147 = Inverse Tangent (2 Input)(1:w389, 2:w388) -> (0:w380:dbl)
              n148 = Add(x=w380, y=3.141592653589793) -> (x+y=w378:dbl)
              n149 = Add(x=w360, y=w362) -> (x+y=w361:dbl[])
              n150 = Insert Into Array(array=w361, index=2, new element=w378) -> (w373:dbl[])
              n151 = case shown="0, Default" w386 {
                tunnel: w381 -> [w400 w403 w406 w409 w412 w415 w418 w421]
                tunnel: w373 -> [w399 w402 w405 w408 w411 w414 w417 w420]
                tunnel: [w398 w401 w404 w407 w410 w413 w416 w419] -> w377
                frame 0, Default {
                  n152 = call "GoTo.vi"("Target"=w399, "Position"=w400) -> ("Output\nVelocity"=w398:dbl[])  [unwired: 8 in, 1 out]
                }
                frame 1 {
                  n153 = call "GoTo.vi"("Target"=w402, "Position"=w403) -> ("Output\nVelocity"=w401:dbl[])  [unwired: 8 in, 1 out]
                }
                frame 2 {
                  n154 = call "GoTo.vi"("Target"=w405, "Position"=w406) -> ("Output\nVelocity"=w404:dbl[])  [unwired: 8 in, 1 out]
                }
                frame 3 {
                  n155 = call "GoTo.vi"("Target"=w408, "Position"=w409) -> ("Output\nVelocity"=w407:dbl[])  [unwired: 8 in, 1 out]
                }
                frame 4 {
                  n156 = call "GoTo.vi"("Target"=w411, "Position"=w412) -> ("Output\nVelocity"=w410:dbl[])  [unwired: 8 in, 1 out]
                }
                frame 5 {
                  n157 = call "GoTo.vi"("Target"=w414, "Position"=w415) -> ("Output\nVelocity"=w413:dbl[])  [unwired: 8 in, 1 out]
                }
                frame 6 {
                  n158 = call "GoTo.vi"("Target"=w417, "Position"=w418) -> ("Output\nVelocity"=w416:dbl[])  [unwired: 8 in, 1 out]
                }
                frame 7 {
                  n159 = call "GoTo.vi"("Target"=w420, "Position"=w421) -> ("Output\nVelocity"=w419:dbl[])  [unwired: 8 in, 1 out]
                }
              }
              n160 = Index Array(array=w377) -> (element #1=w376:dbl, element #2=w375:dbl, element #3=w374:dbl)  [unwired: 3 in]
              n161 = Index Array(array=w373) -> (element #1=w355:dbl, element #2=w354:dbl, element #3=w353:dbl)  [unwired: 3 in]
              n162 = Bundle By Name(cluster=T7 {"dest_x"=0.0, "dest_y"=0.0, "dest_orientation"=0.0, "dest_vel"=0.0} ("Dest"), "dest_x"=w355, "dest_y"=w354, "dest_orientation"=w353, "dest_vel"=0.0) -> (w358:T7)
              n163 = Build Array(w358) -> (w356:T7[])
              n164 = Bundle By Name(cluster=w372, "v_tangent"=w376, "v_normal"=w375, "v_ang"=w374, "Dest"=w356, "dribble"=w352) -> (w371:T3)
            }
            frame False {
              n165 = Select(t=w427, s=w422, f=w426) -> (s? t:f=w425:dbl[])
              n166 = case shown="1" w434 {
                tunnel: w429 -> [w448 w462 w476 w490 w504 w518 w532 w545]
                tunnel: w433 -> [w449 w463 w477 w491 w505 w519 w533 w543]
                tunnel: w435 -> [w447 w461 w475 w489 w503 w517 w531 w547]
                tunnel: w423 -> [w446 w460 w474 w488 w502 w516 w530 w546]
                tunnel: [w445 w459 w473 w487 w501 w515 w529 w544] -> w428
                tunnel: w432 -> [w444 w458 w472 w486 w500 w514 w528 w542]
                tunnel: w431 -> [w443 w457 w471 w485 w499 w513 w527 w541]
                tunnel: w430 -> [w442 w456 w470 w484 w498 w512 w526 w540]
                tunnel: w425 -> [w439 w453 w467 w481 w495 w509 w523 w537]
                tunnel: w424 -> [w437 w451 w465 w479 w493 w507 w521 w535]
                frame 0, Default {
                  n167 = Unbundle By Name(w442) -> ("Attacker.ball-robot Kick"=w441:dbl, "Attacker.CC chute"=w440:dbl)
                  n168 = call "GoToKick.vi"("goleiro?"=w444, "Dribble"=w437, "balls"=w447, "Robot in in"=w448, "Field Size in"=w449, "Target"=w439, "Defender"=TRUE, "D ball - robot"=w441, "AI Parameters"=w442, "Cone de chute"=w440, "Personalidade"=PersonalityEnum."Defender", "Kick Force"=w443, "IA State Input in"=w446) -> ("Robot out"=w445:T3)  [unwired: 3 in, 3 out]
                }
                frame 2 {
                  n169 = Unbundle By Name(w456) -> ("Attacker.ball-robot Kick"=w455:dbl, "Attacker.CC chute"=w454:dbl)
                  n170 = call "GoToKick.vi"("goleiro?"=w458, "Dribble"=w451, "balls"=w461, "Robot in in"=w462, "Field Size in"=w463, "Target"=w453, "Defender"=TRUE, "D ball - robot"=w455, "AI Parameters"=w456, "Cone de chute"=w454, "Personalidade"=PersonalityEnum."Defender", "Kick Force"=w457, "IA State Input in"=w460) -> ("Robot out"=w459:T3)  [unwired: 3 in, 3 out]
                }
                frame 3 {
                  n171 = Unbundle By Name(w470) -> ("Attacker.ball-robot Kick"=w469:dbl, "Attacker.CC chute"=w468:dbl)
                  n172 = call "GoToKick.vi"("goleiro?"=w472, "Dribble"=w465, "balls"=w475, "Robot in in"=w476, "Field Size in"=w477, "Target"=w467, "Defender"=TRUE, "D ball - robot"=w469, "AI Parameters"=w470, "Cone de chute"=w468, "Personalidade"=PersonalityEnum."Defender", "Kick Force"=w471, "IA State Input in"=w474) -> ("Robot out"=w473:T3)  [unwired: 3 in, 3 out]
                }
                frame 4 {
                  n173 = Unbundle By Name(w484) -> ("Attacker.ball-robot Kick"=w483:dbl, "Attacker.CC chute"=w482:dbl)
                  n174 = call "GoToKick.vi"("goleiro?"=w486, "Dribble"=w479, "balls"=w489, "Robot in in"=w490, "Field Size in"=w491, "Target"=w481, "Defender"=TRUE, "D ball - robot"=w483, "AI Parameters"=w484, "Cone de chute"=w482, "Personalidade"=PersonalityEnum."Defender", "Kick Force"=w485, "IA State Input in"=w488) -> ("Robot out"=w487:T3)  [unwired: 3 in, 3 out]
                }
                frame 5 {
                  n175 = Unbundle By Name(w498) -> ("Attacker.ball-robot Kick"=w497:dbl, "Attacker.CC chute"=w496:dbl)
                  n176 = call "GoToKick.vi"("goleiro?"=w500, "Dribble"=w493, "balls"=w503, "Robot in in"=w504, "Field Size in"=w505, "Target"=w495, "Defender"=TRUE, "D ball - robot"=w497, "AI Parameters"=w498, "Cone de chute"=w496, "Personalidade"=PersonalityEnum."Defender", "Kick Force"=w499, "IA State Input in"=w502) -> ("Robot out"=w501:T3)  [unwired: 3 in, 3 out]
                }
                frame 6 {
                  n177 = Unbundle By Name(w512) -> ("Attacker.ball-robot Kick"=w511:dbl, "Attacker.CC chute"=w510:dbl)
                  n178 = call "GoToKick.vi"("goleiro?"=w514, "Dribble"=w507, "balls"=w517, "Robot in in"=w518, "Field Size in"=w519, "Target"=w509, "Defender"=TRUE, "D ball - robot"=w511, "AI Parameters"=w512, "Cone de chute"=w510, "Personalidade"=PersonalityEnum."Defender", "Kick Force"=w513, "IA State Input in"=w516) -> ("Robot out"=w515:T3)  [unwired: 3 in, 3 out]
                }
                frame 7 {
                  n179 = Unbundle By Name(w526) -> ("Attacker.ball-robot Kick"=w525:dbl, "Attacker.CC chute"=w524:dbl)
                  n180 = call "GoToKick.vi"("goleiro?"=w528, "Dribble"=w521, "balls"=w531, "Robot in in"=w532, "Field Size in"=w533, "Target"=w523, "Defender"=TRUE, "D ball - robot"=w525, "AI Parameters"=w526, "Cone de chute"=w524, "Personalidade"=PersonalityEnum."Defender", "Kick Force"=w527, "IA State Input in"=w530) -> ("Robot out"=w529:T3)  [unwired: 3 in, 3 out]
                }
                frame 1 {
                  n181 = Unbundle By Name(w540) -> ("Attacker.ball-robot Kick"=w539:dbl, "Attacker.CC chute"=w538:dbl)
                  n182 = call "GoToKick.vi"("goleiro?"=w542, "Dribble"=w535, "balls"=w547, "Robot in in"=w545, "Field Size in"=w543, "Target"=w537, "Defender"=TRUE, "D ball - robot"=w539, "AI Parameters"=w540, "Cone de chute"=w538, "Personalidade"=PersonalityEnum."Defender", "Kick Force"=w541, "IA State Input in"=w546) -> ("Robot out"=w544:T3)  [unwired: 3 in, 3 out]
                }
              }
            }
          }
        }
      }
      n183 = feedback-in #1(w95) -> ()
    }
  }
  "Robot out" <- w5
  "Pos Centers Back" <- w4
